vi "Configure Current Slew Negative.vi"(7 "Channel":i32(ring)=1 items=["Channel 1"=1, "Channel 2"=2, "Channel 3"=3, "Channel 4"=4, "Channel 5"=5, "Channel 6"=6, "Channel 7"=7, "Channel 8"=8, "Channel 8"=9, "Channel 10"=10, "Channel 11"=11, "Channel 12"=12, "Channel 13"=13, "Channel 14"=14, "Channel 15"=15, "Channel 16"=16], 8 "error in":errorcluster, 10 "Slew":dbl min=0.0, 11 "VISA resource name":refnum<visa-resource-name>) -> (0 "error out":errorcluster, 3 "VISA resource name out":refnum<visa-resource-name>)   [LabVIEW 2020, in "IT-M3400.lvlib"]
doc: "This command sets the current drop slope of the source output.\n<b>Slew</b>\nMIN-MAX"
uses:
  IT-M3400.lvlib
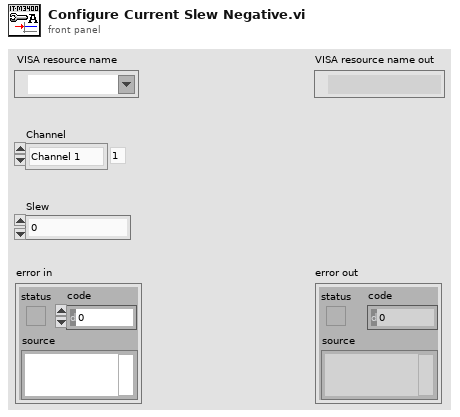
[diagram p1: front panel]
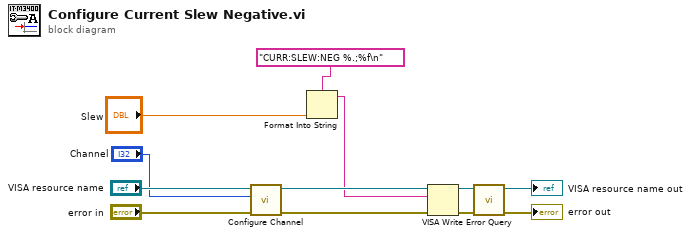
[diagram p0: block diagram]
diagram:
  n1 = call "Configure Channel.vi"("error in"="error in", "Channel"="Channel", "VISA resource name"="VISA resource name") -> ("error out"=w4:errorcluster, "VISA resource name out"=w5:refnum<visa-resource-name>)  [unwired: 7 in]
  n2 = Format Into String(format string="CURR:SLEW:NEG %.;%f\n", "Slew") -> (resulting string=w2:string)  [unwired: 2 in, 1 out]
  n3 = VISA Write(VISA resource name=w5, write buffer=w2, error in (no error)=w4) -> (VISA resource name out=w9:refnum<visa-resource-name>, error out=w10:errorcluster)  [unwired: 1 out]
  n4 = call "Error Query.vi"("error in"=w10, "VISA resource name"=w9) -> ("error out"=→"error out":errorcluster, "VISA resource name out"=→"VISA resource name out":refnum<visa-resource-name>)  [unwired: 7 in, 1 out]
